vi "test-trapezoid-profile-reaches-goal.vi"() -> ()   [LabVIEW 2019]
uses:
  <vilib>/Rock Robotics/WPI/ThirdParty/JAS_Junk/TrajLib/TRAPEZOID_PROFILE_STATE.ctl
  <vilib>/Rock Robotics/WPI/ThirdParty/JAS_Junk/TrajLib/TrapProfile_ShouldFlipAcceleration.vi
  <vilib>/Rock Robotics/WPI/ThirdParty/JAS_Junk/TrajLib/TrapProfile_Direct.vi
  <vilib>/Rock Robotics/WPI/ThirdParty/JAS_Junk/TrajLib/Trajectory_Library.lvlib
panel:
  out "State":T1 {"Velocity" format="%16_6e"; "Position" format="%16_6e"}
  out "Waveform Chart":T2(graph)
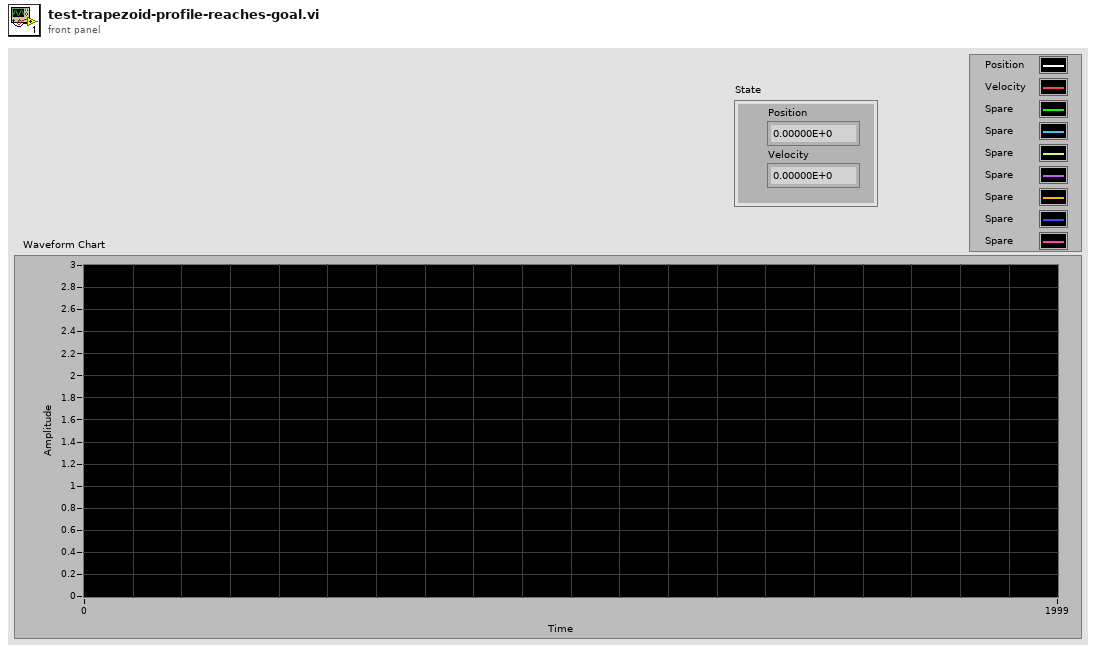
[diagram p1: front panel]
types:
  T1 = typedef "Trajectory_Library.lvlib/TRAPEZOID_PROFILE_STATE.ctl" = cluster{"Position":dbl, "Velocity":dbl}
  T2 = cluster{dbl, dbl, "Output":dbl, "Output":dbl, "Output":dbl, "Output":dbl, "Output":dbl, "Output":dbl, "Output":dbl}
  T3 = typedef "Trajectory_Library.lvlib/TRAPEZOID_PROFILE_CONSTRAINT.ctl" = cluster{"MaxVelocity":dbl, "MaxAcceleration":dbl}
  T4 = typedef "Trajectory_Library.lvlib/TRAPEZOID_PROFILE.ctl" = cluster{"EndAccel":dbl, "EndFullSpeed":dbl, "EndDecel":dbl, "Direction":i32, "Constraints":T3, "Initial":T1, "Goal":T1}
  T5 = cluster{"Position":dbl, "Velocity":dbl, "Velocity":dbl, "Velocity":dbl, "Velocity":dbl, "Velocity":dbl, "Velocity":dbl, "Velocity":dbl, "Velocity":dbl}
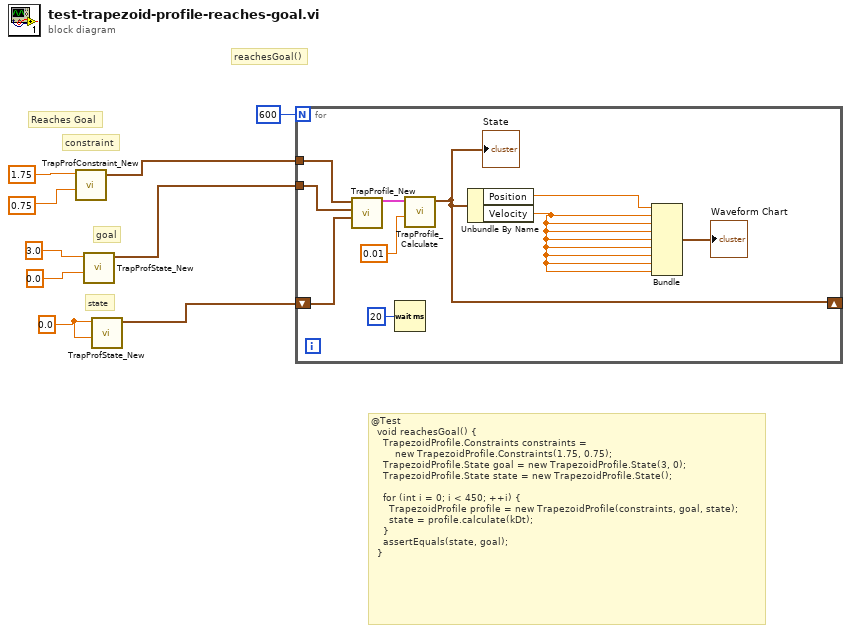
[diagram p0: block diagram]
diagram:
  w7 = 0.0 ("Position")
  # "@Test\n  void reachesGoal() {\n    TrapezoidProfile.Constraints constraints =\n        new TrapezoidProfile.Constraints(1.75, 0.75);\n    TrapezoidProfile.State goal = new TrapezoidProfile.State(3, 0);\n    TrapezoidProfile.State state = new TrapezoidProfile.State();\n\n    for (int i = 0; i < 450; ++i) {\n      TrapezoidProfile profile = new TrapezoidProfile(constraints, goal, state);\n      state = profile.calculate(kDt);\n    }\n    assertEquals(state, goal);\n  }"
  # "reachesGoal()"
  # "goal"
  # "state"
  # "Reaches Goal"
  # "constraint"
  n1 = call <vilib>:"TrapProfConstraint_New.vi"("Max Accel"=0.75, "Max Speed (M/S)"=1.75) -> ("TRAPEZOID_PROFILE_CONSTRAINT"=w3:T3)  [unwired: 9 in]
  n2 = call <vilib>:"TrapProfState_New.vi"("Velocity"=0.0, "Position"=3.0) -> ("TRAPEZOID_PROFILE_STATE"=w2:T1)  [unwired: 9 in]
  n3 = call <vilib>:"TrapProfState_New.vi"("Velocity"=w7, "Position"=w7) -> ("TRAPEZOID_PROFILE_STATE"=w1:T1)  [unwired: 9 in]
  n4 = for {
    N: 600 -> [_]
    tunnel: w3 -> [w15]
    tunnel: w2 -> [w14]
    shift-right: [w13] -> _
    shift-left: w1 -> [w10]
    n5 = call <vilib>:"TrapProfile_New.vi"("Initial"=w10, "Goal"=w14, "Constraints"=w15) -> ("TRAPEZOID_PROFILE"=w12:T4)  [unwired: 8 in]
    n6 = Wait (ms)(milliseconds to wait=u32 20) -> ()  [unwired: 1 out]
    n7 = call <vilib>:"TrapProfile_Calculate.vi"("Time"=0.01, "TRAPEZOID_PROFILE"=w12) -> ("State"=w13:T1)  [unwired: 9 in]
    "State" <- w13
    n8 = Unbundle By Name(w13) -> ("Position"=w16:dbl, "Velocity"=w17:dbl)
    n9 = Bundle("Position"=w16, "Velocity"=w17, "Velocity"=w17, "Velocity"=w17, "Velocity"=w17, "Velocity"=w17, "Velocity"=w17, "Velocity"=w17, "Velocity"=w17) -> (→"Waveform Chart":T5)  [unwired: 1 in]
  }
